vi "Configure Arb Frequency [AF].vi"(8 "error in (no error)":errorcluster, 9 "frequency (0.0 Hz)":dbl[unit] format="%.3f", 10 "channel name (\"CHANNEL1\")":string="CHANNEL1", 11 "CS++Fgen in":refnum<class "CS++Fgen.lvclass">) -> (0 "error out":errorcluster, 3 "CS++Fgen out":refnum<class "CS++Fgen.lvclass">)   [LabVIEW 2015, in "CS++Fgen.lvlib" / "CS++Fgen.lvclass"]
doc: "This VI configures the rate at which the function generator produces an entire cycle of an arbitrary waveform on a channel.\n \nNotes:\n\n(1) This VI is part of the IviFgenArbFrequency [AF] extension group."
uses:
  CS++Fgen.lvclass
  CSPP_Core/Classes/CS++ProcessVariables/ProcessVariable/PV.lvclass
  PV-Enum-n.ctl
  CSPP_Core/Classes/CS++ProcessVariables/ProcessVariable/PV.lvclass/PV.ctl
  CS++Fgen.lvclass/CS++Fgen.ctl
  CSPP_Core/Classes/CS++ProcessVariables/ProcessVariable/Write Data.vi
  CSPP_Core/Classes/CS++ProcessVariables/ProcessVariable/Write Timestamp.vi
  CSPP_Core/Classes/CS++ProcessVariables/ProcessVariable/Write Quality.vi
  CSPP_Core/Classes/CS++ProcessVariables/ProcessVariable/Write status.vi
  CSPP_Core/Classes/CS++ProcessVariables/PVConnection/PVConnection.lvclass
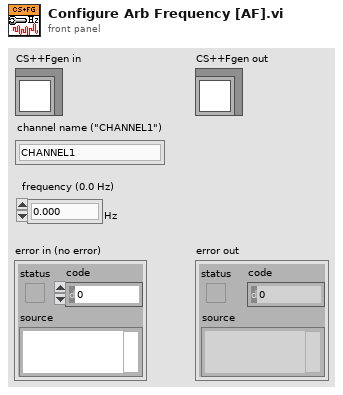
[diagram p1: front panel]
types:
  T1 = typedef "CS++Fgen.lvlib/CS++Fgen.lvclass/PV-Enum-n.ctl" = enum16{"Amplitude", "Arb-Frequency", "DCOffset", "Frequency", "OutputImpedance", "StartPhase", "AdvancedTriggerSlope", "AM-Source", "BurstCount", "FM-Source", "OperationMode", "ResumeTriggerSlope", "StartTriggerSlope", "StopTriggerSlope", "Waveform", "TriggerSource", "AM-Enabled", "ChannelEnabled", "FM-Enabled", "AdvancedTriggerSource", "ResumeTriggerSource", "StartTriggerSource", "StopTriggerSource"}
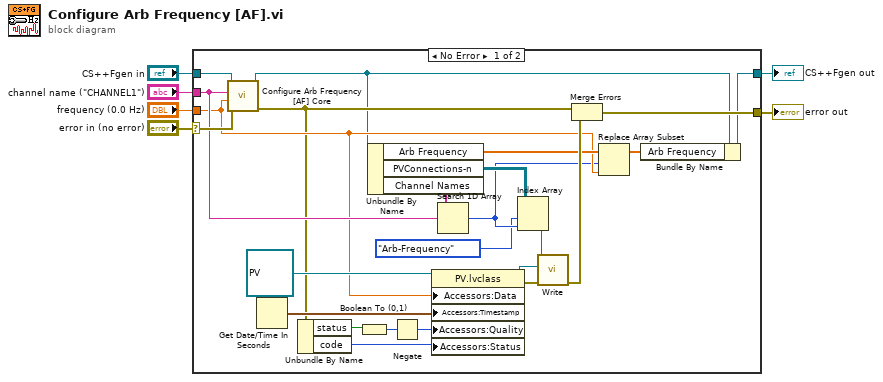
[diagram p0: block diagram]
diagram:
  n1 = case shown="No Error" "error in (no error)" {
    selector: "error in (no error)" -> [w29 w32]
    tunnel: [w11 w32] -> w5
    tunnel: [w9 w31] -> w3
    tunnel: "CS++Fgen in" -> [w30 w31]
    tunnel: "frequency (0.0 Hz)" -> [w13 _]
    tunnel: "channel name (\"CHANNEL1\")" -> [w14 _]
    frame No Error {
      n2 = call-dynamic "Configure Arb Frequency [AF] Core.vi"("error in (no error)"=w29, "frequency (0.0 Hz)"=w13, "channel name (\"CHANNEL1\")"=w14, "CS++Fgen in"=w30) -> ("error out"=w12:errorcluster, "CS++Fgen out"=w10:refnum<class "CS++Fgen.lvclass">)  [unwired: 6 in]
      n3 = Get Date/Time In Seconds() -> (seconds since 1Jan1904=w28:timestamp)
      n4 = Unbundle By Name(w12) -> ("status"=w20:bool, "code"=w18:i32)
      n5 = Boolean To (0,1)(Boolean=w20) -> (0, 1=w19:i16)
      n6 = Unbundle By Name(w10) -> ("Arb Frequency"=w16:dbl[unit][], "PVConnections-n"=w23:refnum<class "PVConnection.lvclass">[][], "Channel Names"=w24:string[])
      n7 = Negate(x=w19) -> (-x=w17:i16)
      n8 = property class="PV.lvclass"(reference=refnum<class "PV.lvclass"> refnum ("PV"), "Accessors:Data"=w13, "Accessors:Timestamp"=w28, "Accessors:Quality"=w17, "Accessors:Status"=w18) -> (reference out=w25:refnum<class "PV.lvclass">, error out=w26:errorcluster)  [unwired: 1 in]
      n9 = Search 1D Array(1D array=w24, element=w14) -> (index of element=w8:i32)  [unwired: 1 in]
      n10 = Index Array(array=w23, index (row)=PV-Enum-n."Arb-Frequency" ("PV-Enum-n"), index (col)=w8) -> (element=w22:refnum<class "PVConnection.lvclass">)
      n11 = call "Write.vi"("error in (no error)"=w26, "PV"=w25, "PVConnection in"=w22) -> ("error out"=w21:errorcluster)  [unwired: 7 in, 1 out]
      n12 = Merge Errors(w12, w21) -> (w11:errorcluster)
      n13 = Replace Array Subset(array=w16, new element=w13, index=w8) -> (w15:dbl[unit][])
      n14 = Bundle By Name(cluster=w10, "Arb Frequency"=w15) -> (w9:refnum<class "CS++Fgen.lvclass">)
    }
    frame Error {
    }
  }
  "error out" <- w5
  "CS++Fgen out" <- w3
